vi "subvi_Connect.vi"(8 "에러":errorcluster caption="에러 입력", 9 "baud rate":u32, 10 "unit ID":u8, 11 "VISA 참조 번호 입력":refnum<visa-resource-name>) -> (0 "에러 출력":errorcluster, 2 "register values":u16[](array[numeric]), 3 "Modbus Master 출력":refnum<class "Modbus Master.lvclass">)   [LabVIEW 2016]
uses:
  <vilib>/NI/Modbus Library/API/Master/Modbus Master.lvclass
  <vilib>/NI/Modbus Library/API/Wrapper/Create Serial Master.vi
  <vilib>/NI/Modbus Library/API/Wrapper/API Main.lvlib
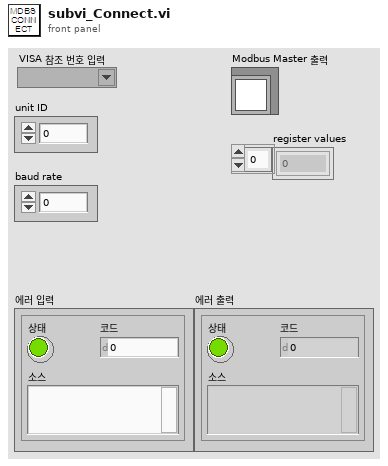
[diagram p1: front panel]
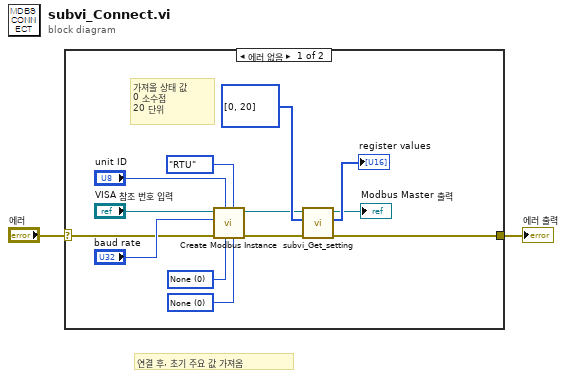
[diagram p0: block diagram]
diagram:
  # "연결 후, 초기 주요 값 가져옴"
  n1 = case shown="에러 없음" "에러" {
    selector: "에러" -> [w4 w16]
    tunnel: [w3 w16] -> w1
    frame No Error {
      w11 = u16 0 items=["None", "XON/XOFF", "RTS/CTS", "XON/XOFF & RTS/CTS", "DTR/DSR", "XON/XOFF & DTR/DSR"] ("flow control (none)")
      w10 = u16 0 items=["None", "Odd", "Even", "Mark", "Space"] ("parity (even)")
      # "가져올 상태 값\n0 소수점\n20 단위"
      n2 = call-poly <vilib>:"Create Modbus Instance.vi"("flow control (none)"=w11, "serial type"=enum16{"RTU", "ASCII"}."RTU", "parity (even)"=w10, "unit ID"="unit ID", "error in"=w4, "baud rate"="baud rate", "VISA resource name"="VISA 참조 번호 입력") -> ("error out"=w5:errorcluster, "serial master instance"=w13:refnum<class "Modbus Master.lvclass">)  [unwired: 3 in]
      n3 = call "subvi_Get_setting.vi"("에러 입력(에러 없음)"=w5, "Input adress"=u16[] [0, 20], "Modbus Master 입력"=w13) -> ("에러 출력"=w3:errorcluster, "register values"=→"register values":u16[], "Modbus Master 출력"=→"Modbus Master 출력":refnum<class "Modbus Master.lvclass">)  [unwired: 6 in]
    }
    frame Error {
    }
  }
  "에러 출력" <- w1
